vi "Register Hot And Cold Source Unit View.vi"(11 "Message Enqueuer in":refnum<class "Message Enqueuer.lvclass">) -> (3 "Message Enqueuer out":refnum<class "Message Enqueuer.lvclass">)   [LabVIEW 2013]
uses:
  <vilib>/ActorFramework/Message Enqueuer/Message Enqueuer.lvclass
  <vilib>/ActorFrameworkMVC/View Observer/Registration Message/Registration Message.lvclass
  <vilib>/ActorFrameworkMVC/View Observer/Data Message/Data Message.lvclass
  Models/Hot And Cold Source Unit Model Messages/Register Initialize Hot And Cold Source Unit Msg/Register Initialize Hot And Cold Source Unit Msg.lvclass
  Views/Hot And Cold Source Unit View Messages/Conceret Initialize Hot And Cold Source Unit Msg/Conceret Initialize Hot And Cold Source Unit Msg.lvclass
  Views/Hot And Cold Source Unit View Messages/Conceret Test Node Map Msg/Conceret Test Node Map Msg.lvclass
  Models/Hot And Cold Source Unit Model Messages/Register Test Node Map Msg/Register Test Node Map Msg.lvclass
  Models/Hot And Cold Source Unit Model Messages/Conceret Results Msg/Conceret Results Msg.lvclass
  Models/Hot And Cold Source Unit Model Messages/Register Results Msg/Register Results Msg.lvclass
  <vilib>/ActorFrameworkMVC/UI Controller Messages/Subscribe View to Model Msg/Subscribe View to Model Msg.lvclass/Subscribe View to Model Msg.ctl
  <vilib>/ActorFramework/Message Enqueuer/Message Enqueuer.lvclass/Message Enqueuer.ctl
  <vilib>/ActorFramework/Message Enqueuer/Enqueue.vi
  <vilib>/ActorFramework/Message Priority Queue/Priority Enqueue.vi
  <vilib>/ActorFrameworkMVC/UI Controller Messages/Subscribe View to Model Msg/Subscribe View to Model Msg.lvclass
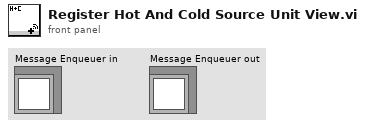
[diagram p1: front panel]
types:
  T1 = cluster{"Registration Message":string, "Data Message":string}[]
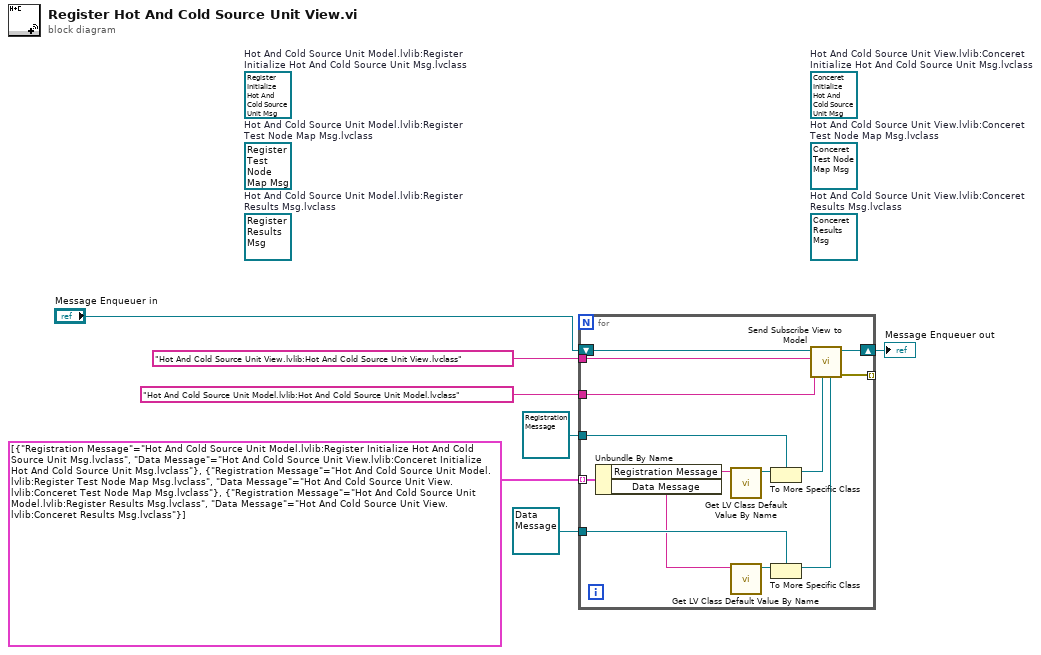
[diagram p0: block diagram]
diagram:
  (unwired) refnum<class "Register Results Msg.lvclass"> refnum  # Hot And Cold Source Unit Model.lvlib:Register Results Msg.lvclass
  (unwired) refnum<class "Conceret Results Msg.lvclass"> refnum  # Hot And Cold Source Unit View.lvlib:Conceret Results Msg.lvclass
  (unwired) refnum<class "Register Test Node Map Msg.lvclass"> refnum  # Hot And Cold Source Unit Model.lvlib:Register Test Node Map Msg.lvclass
  (unwired) refnum<class "Conceret Test Node Map Msg.lvclass"> refnum  # Hot And Cold Source Unit View.lvlib:Conceret Test Node Map Msg.lvclass
  (unwired) refnum<class "Conceret Initialize Hot And Cold Source Unit Msg.lvclass"> refnum  # Hot And Cold Source Unit View.lvlib:Conceret Initialize Hot And Cold Source Unit Msg.lvclass
  (unwired) refnum<class "Register Initialize Hot And Cold Source Unit Msg.lvclass"> refnum  # Hot And Cold Source Unit Model.lvlib:Register Initialize Hot And Cold Source Unit Msg.lvclass
  n1 = for {
    tunnel: "Hot And Cold Source Unit View.lvlib:Hot And Cold Source Unit View.lvclass" ("View Name") -> [w20]
    tunnel: "Hot And Cold Source Unit Model.lvlib:Hot And Cold Source Unit Model.lvclass" ("Model Name") -> [w19]
    shift-right: [w18] -> w7
    shift-left: "Message Enqueuer in" -> [w21]
    tunnel: refnum<class "Registration Message.lvclass"> refnum ("Registration Message") -> [w15]
    tunnel: refnum<class "Data Message.lvclass"> refnum ("Data Message") -> [w14]
    tunnel: T1 [{"Registration Message"="Hot And Cold Source Unit Model.lvlib:Register Initialize Hot And Cold Source Unit Msg.lvclass", "Data Message"="Hot And Cold Source Unit View.lvlib:Conceret Initialize Hot And Cold Source Unit Msg.lvclass"}, {"Registration Message"="Hot And Cold Source Unit Model.lvlib:Register Test Node Map Msg.lvclass", "Data Message"="Hot And Cold Source Unit View.lvlib:Conceret Test Node Map Msg.lvclass"}, {"Registration Message"="Hot And Cold Source Unit Model.lvlib:Register Results Msg.lvclass", "Data Message"="Hot And Cold Source Unit View.lvlib:Conceret Results Msg.lvclass"}] -> [w13] mode=indexing
    tunnel: [w8] -> _ mode=indexing
    n2 = Unbundle By Name(w13) -> ("Registration Message"=w10:string, "Data Message"=w9:string)
    n3 = call <vilib>:"Get LV Class Default Value By Name.vi"("class name"=w10) -> ("object"=w17:refnum<class>)  [unwired: 9 in, 1 out]
    n4 = call <vilib>:"Get LV Class Default Value By Name.vi"("class name"=w9) -> ("object"=w16:refnum<class>)  [unwired: 9 in, 1 out]
    n5 = To More Specific Class(target class=w15, reference=w17) -> (specific class reference=w12:refnum<class "Registration Message.lvclass">)  [unwired: 1 in, 1 out]
    n6 = To More Specific Class(target class=w14, reference=w16) -> (specific class reference=w11:refnum<class "Data Message.lvclass">)  [unwired: 1 in, 1 out]
    n7 = call <vilib>:"Send Subscribe View to Model.vi"("Data Message"=w11, "Registration Message"=w12, "Model Name"=w19, "View Name"=w20, "Message Enqueuer"=w21) -> ("error out"=w8:errorcluster, "Message Enqueuer out"=w18:refnum<class "Message Enqueuer.lvclass">)  [unwired: 5 in]
  }
  "Message Enqueuer out" <- w7
